vi "Teleop.vi"(10 "Match Info":T1={"Autonomous Elapsed Seconds"=0.0, "TeleOp Elapsed Seconds"=0.0, "Disabled Elapsed Seconds"=0.0, "Visited Autonomous"=FALSE, "Visited TeleOp"=FALSE, "Visited Disabled"=FALSE, "Autonomous Settings"={"Autonomous Style"=enum."Independent", "VI Refnum"=refnum}}, 11 "Call Context":T2) -> ()   [LabVIEW 2020]
doc: "This VI is called for each TeleOp packet received from the DS where the robot is not disabled. It is often used to read from the joysticks and update I/O or to update setpoints for timed control loops. It should complete and return within 20 milliseconds or it may miss DS packets."
uses:
  <vilib>/Rock Robotics/WPI/DriverStation/WPI_DriverStationDerivedRobotMode.ctl
  <vilib>/Rock Robotics/WPI/DriverStation/WPI_DriverStationMatch Info.ctl
  <vilib>/Rock Robotics/WPI/ThirdParty/Phoenix-LabVIEW/Motor Controller/Controls/CTRE_Phoenix_MotorControl_NeutralMode.ctl
  <vilib>/Rock Robotics/WPI/RobotDrive/WPI_RobotDriveDevRef.ctl
  <vilib>/Rock Robotics/WPI/MotorControl/WPI_MotorControlDeviceRef.ctl
  <vilib>/Rock Robotics/WPI/MotorControl/WPI_MotorControlType.ctl
  <vilib>/Rock Robotics/SystemInterfaces/DIO/FPGA_DIOPWMChannel.ctl
  <vilib>/Rock Robotics/WPI/PWM/WPI_PWMDeadband.ctl
  <vilib>/Rock Robotics/SystemInterfaces/DIO/FPGA_DIOChannel.ctl
  <vilib>/Rock Robotics/WPI/SafetyOutput/WPI_SafetyOutputConfigMenu.ctl
  <vilib>/Rock Robotics/WPI/Utilities/WPI_GetSetVariantRefNum.vi
  V1_nauru_2023_06_22/Global 1.vi
panel:
  out "FlagGarra":bool
  out "flagModoReto":bool
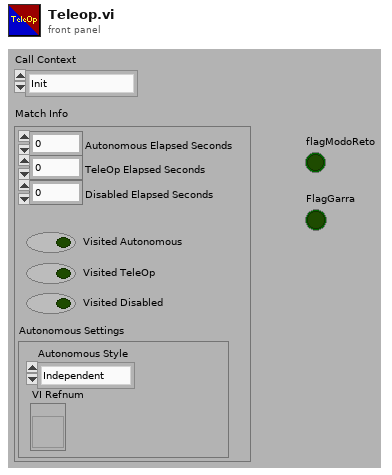
[diagram p1: front panel]
types:
  T1 = typedef "WPI_DriverStationMatch Info.ctl" = cluster{"Autonomous Elapsed Seconds":dbl, "TeleOp Elapsed Seconds":dbl, "Disabled Elapsed Seconds":dbl, "Visited Autonomous":bool, "Visited TeleOp":bool, "Visited Disabled":bool, "Autonomous Settings":cluster{"Autonomous Style":enum16{"Iterative", "Independent"}, "VI Refnum":refnum<vi>}}
  T2 = typedef "WPI_DriverStationDerivedRobotMode.ctl" = enum16{"Init", "Execute", "Stop"}
  T3 = typedef "WPI_SafetyOutputConfigMenu.ctl" = enum16{"Enable", "Disable"}
  T4 = typedef "WPI_RobotDriveDevRef.ctl" = cluster{"DevStatus":errorcluster, "Motors[]":T5[], "Square Inputs":bool, "Max Output":dbl}
  T5 = typedef "WPI_MotorControlDeviceRef.ctl" = cluster{"DeviceStatus":errorcluster, "Type":T6, "PWM":cluster{"PWM Channel":T7, "DeadBand":T8}, "CAN":cluster{"Device Number":u8, "SetOutput VI Ref":variant, "GetOutput VI Ref":variant, "Enable VI Ref":variant, "Disable VI Ref":variant, "Data":variant}, "Invert":bool, "DIO PWM":cluster{"PWM \"Enable\" Channel":T7, "DIOChannel":T9, "PWM Rate":dbl}}
  T6 = typedef "WPI_MotorControlType.ctl" = enum16{"PWM", "CAN", "DIO PWM"}
  T7 = typedef "FPGA_DIOPWMChannel.ctl" = enum8{"PWM 0", "PWM 1", "PWM 2", "PWM 3", "PWM 4", "PWM 5", "PWM 6", "PWM 7", "PWM 8", "PWM 9", "PWM MXP 0", "PWM MXP 1", "PWM MXP 2", "PWM MXP 3", "PWM MXP 4", "PWM MXP 5", "PWM MXP 6", "PWM MXP 7", "PWM MXP 8", "PWM MXP 9", "Invalid"}
  T8 = typedef "WPI_PWMDeadband.ctl" = cluster{"Name":string, "maxPositivePwm":i32, "minPositivePwm":i32, "centerPwm":i32, "maxNegativePwm":i32, "minNegativePwm":i32, "angularRange":u16}
  T9 = typedef "FPGA_DIOChannel.ctl" = enum8{"DIO 0", "DIO 1", "DIO 2", "DIO 3", "DIO 4", "DIO 5", "DIO 6", "DIO 7", "DIO 8", "DIO 9", "DIO MXP 0", "DIO MXP 1", "DIO MXP 2", "DIO MXP 3", "DIO MXP 4", "DIO MXP 5", "DIO MXP 6", "DIO MXP 7", "DIO MXP 8", "DIO MXP 9", "DIO MXP 10", "DIO MXP 11", "DIO MXP 12", "DIO MXP 13", "DIO MXP 14", "DIO MXP 15", "SPI Port CS1", "SPI Port CS2", "SPI Port CS3", "SPI Port MISO", "SPI Port MOSI", "Invalid"}
  T10 = typedef "CTRE_Phoenix_MotorControl_NeutralMode.ctl" = enum8{"EEPROMSetting", "Override to Coast", "Override to Brake"}
  T11 = typedef "WPI_JoystickDevRef.ctl" = cluster{"Device":T12}
  T12 = typedef "WPI_JoystickDeviceEnum.ctl" = enum16{"USB 0", "USB 1", "USB 2", "USB 3", "USB 4", "USB 5"}
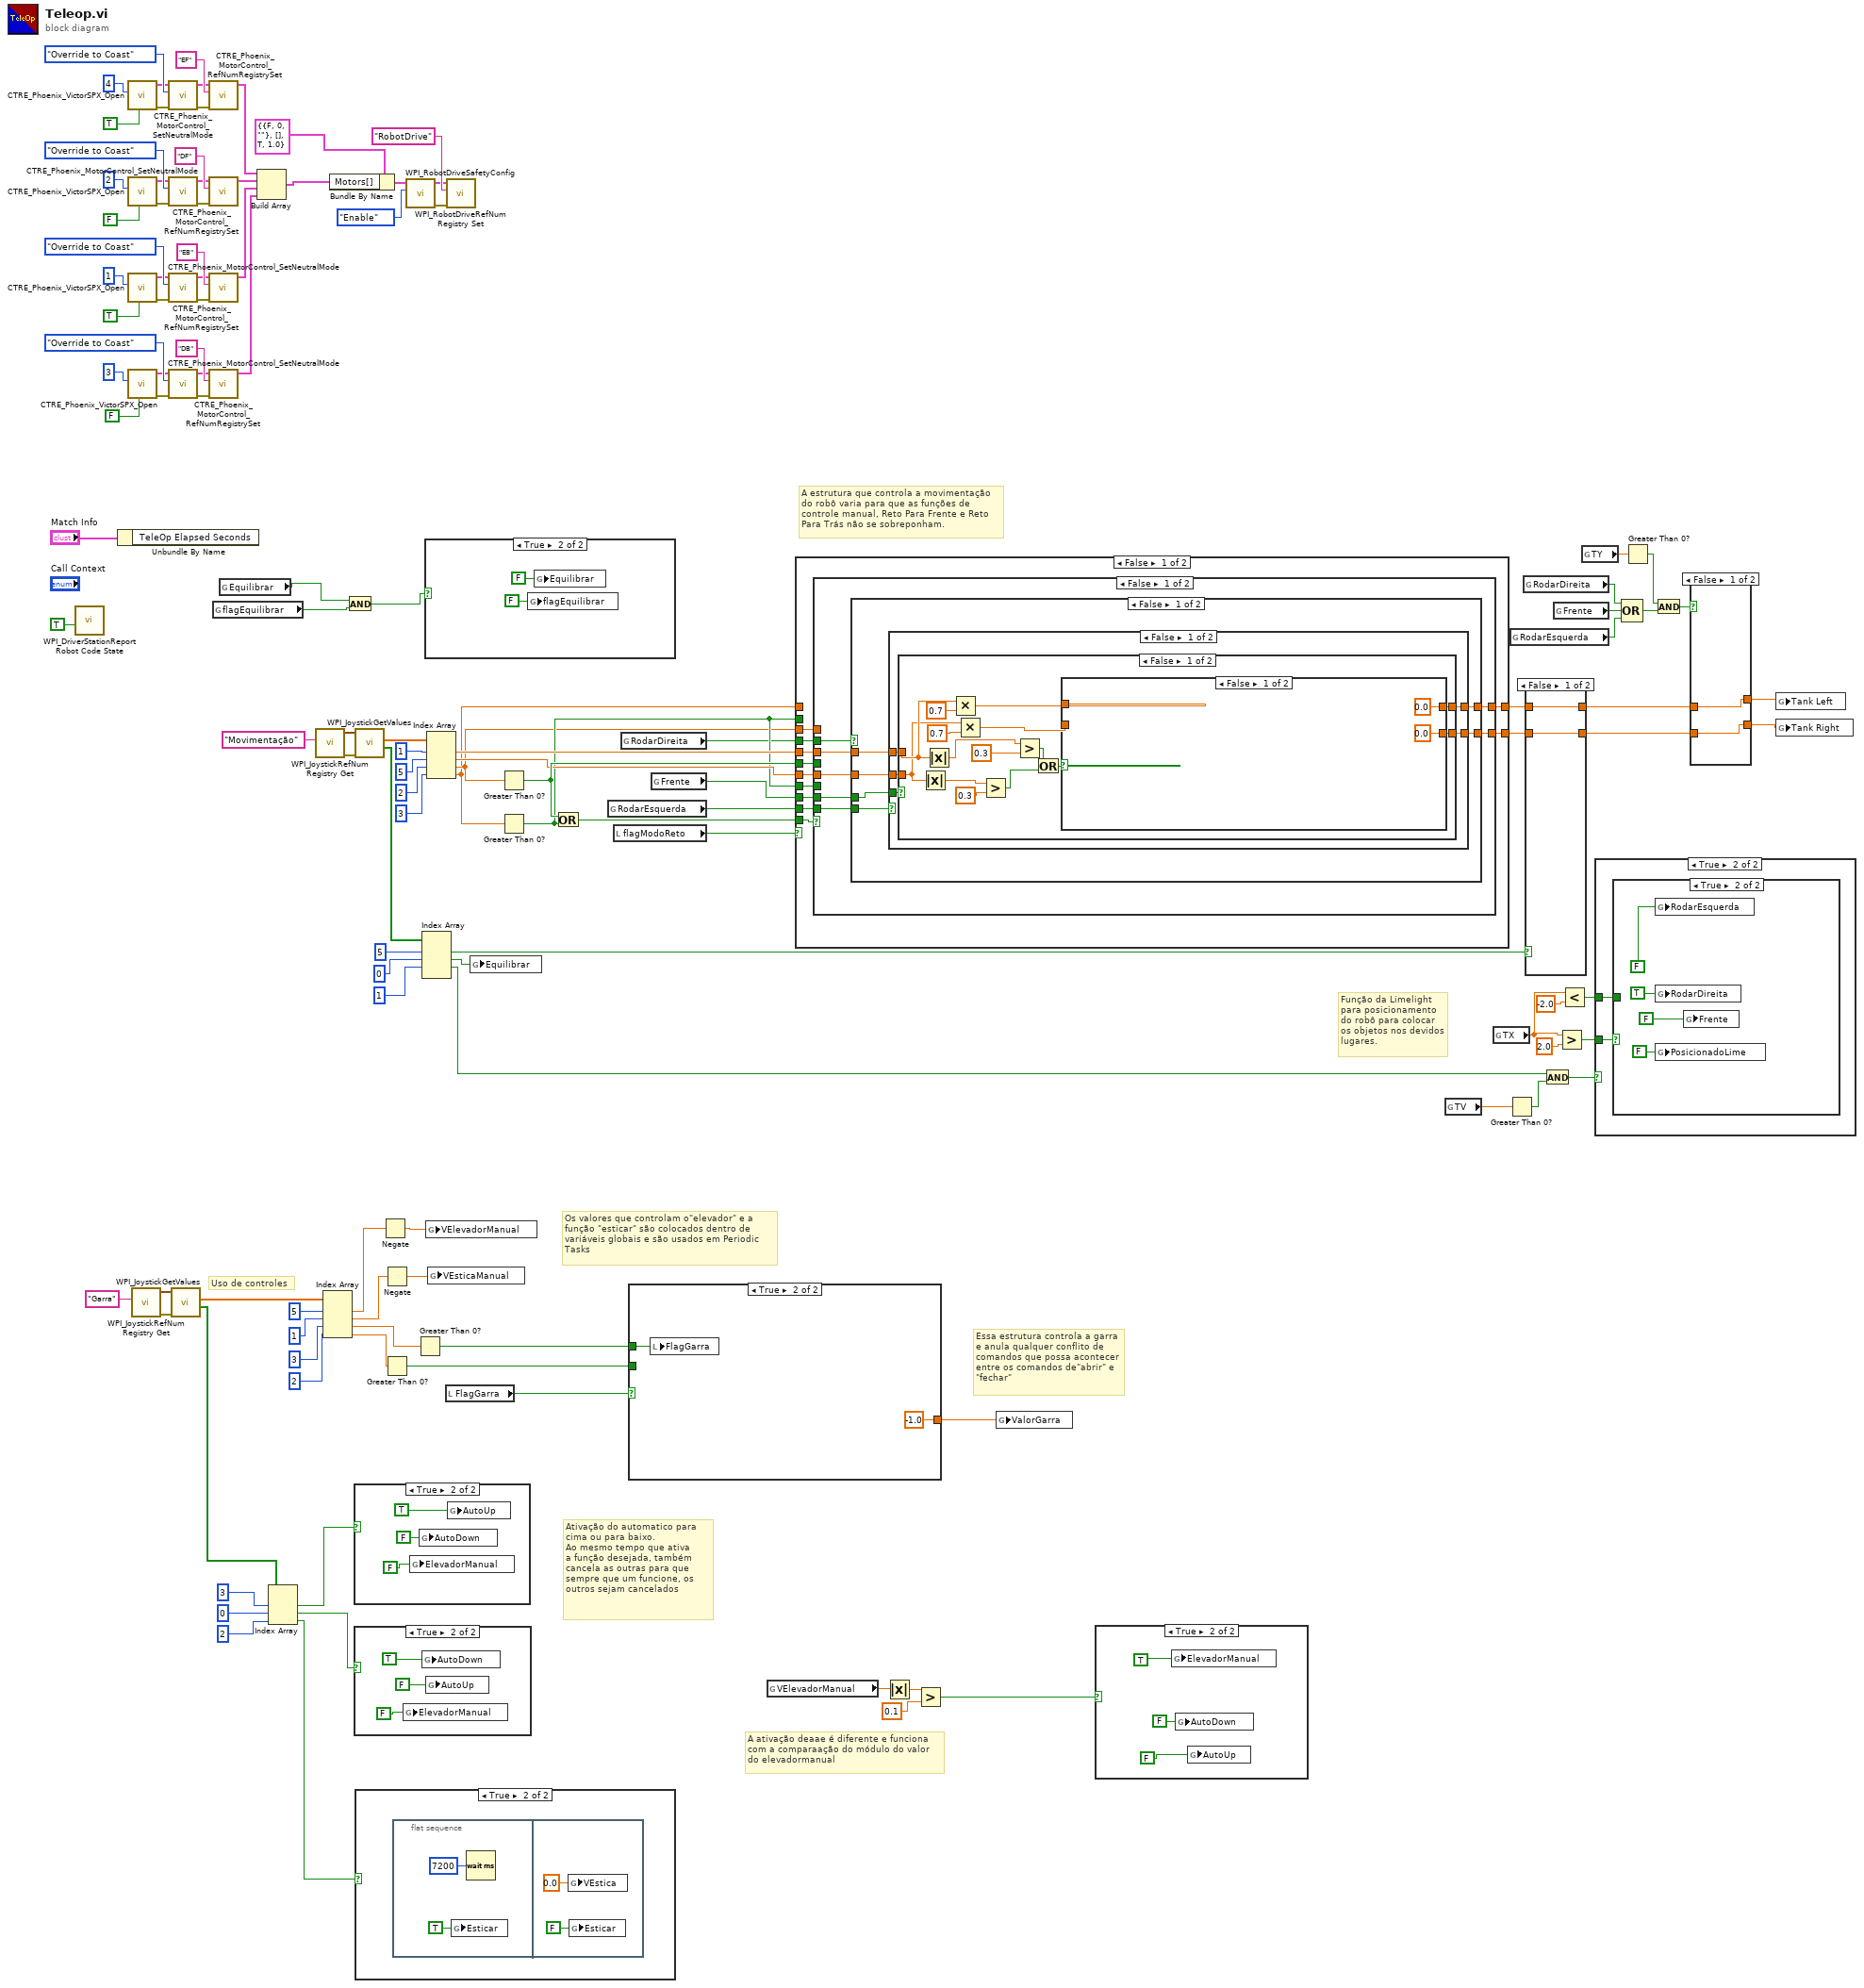
[diagram p0: block diagram]
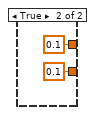
[diagram p4: hidden frame]
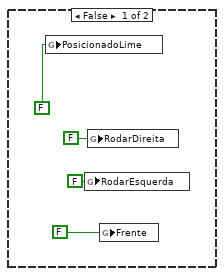
[diagram p5: hidden frame]
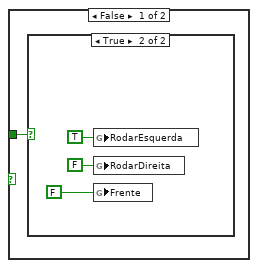
[diagram p6: hidden frame]
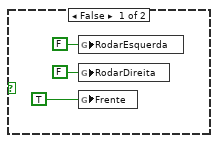
[diagram p7: hidden frame]
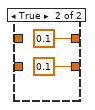
[diagram p8: hidden frame]
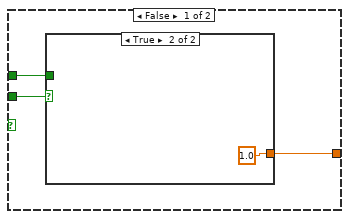
[diagram p12: hidden frame]
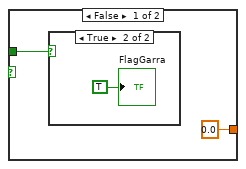
[diagram p13: hidden frame]
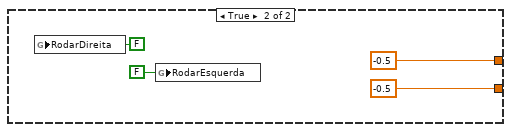
[diagram p16: hidden frame]
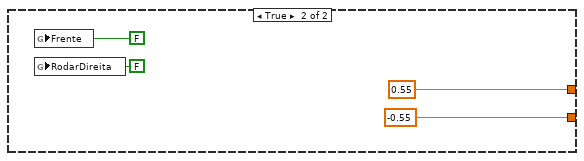
[diagram p17: hidden frame]
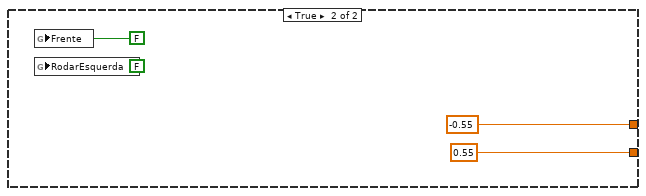
[diagram p18: hidden frame]
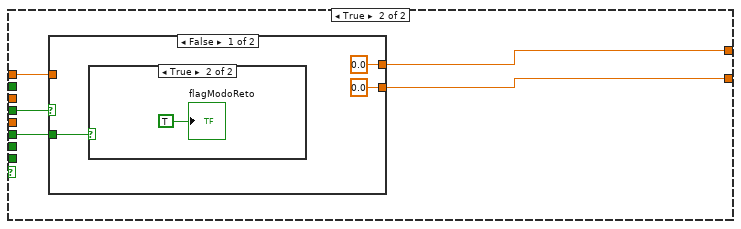
[diagram p19: hidden frame]
diagram:
  # "Função da Limelight para posicionamento do robô para colocar os objetos nos devidos lugares."
  # "Uso de controles"
  # "Essa estrutura controla a garra e anula qualquer conflito de comandos que possa acontecer entre os comandos de\"abrir\" e \"fechar\""
  # "Os valores que controlam o\"elevador\" e a função \"esticar\" são colocados dentro de variáveis globais e são usados em Periodic Tasks"
  # "A ativação deaae é diferente e funciona com a comparaação do módulo do valor do elevadormanual"
  # "A estrutura que controla a movimentação do robô varia para que as funções de controle manual, Reto Para Frente e Reto Para Trás não se sobreponham."
  # "Ativação do automatico para\ncima ou para baixo.\nAo mesmo tempo que ativa\na função desejada, também\ncancela as outras para que \nsempre que um funcione, os \noutros sejam cancelados"
  n1 = call <vilib>:"WPI_DriverStationReport Robot Code State.vi"("TeleOp"=TRUE ("Autonomous")) -> ()  [unwired: 10 in, 1 out]
  n2 = Unbundle By Name("Match Info") -> ()  [unwired: 1 out]
  n3 = call <vilib>:"CTRE_Phoenix_VictorSPX_Open.vi"("Invert"=TRUE, "Device Number"=u8 4) -> ("error out"=w8:errorcluster, "PhoenixMotorControlDevRef"=w9:T5)  [unwired: 8 in]
  n4 = call <vilib>:"CTRE_Phoenix_VictorSPX_Open.vi"("Invert"=FALSE, "Device Number"=u8 2) -> ("error out"=w16:errorcluster, "PhoenixMotorControlDevRef"=w17:T5)  [unwired: 8 in]
  n5 = call <vilib>:"CTRE_Phoenix_VictorSPX_Open.vi"("Invert"=TRUE, "Device Number"=u8 1) -> ("error out"=w24:errorcluster, "PhoenixMotorControlDevRef"=w25:T5)  [unwired: 8 in]
  n6 = call <vilib>:"CTRE_Phoenix_VictorSPX_Open.vi"("Invert"=FALSE, "Device Number"=u8 3) -> ("error out"=w32:errorcluster, "PhoenixMotorControlDevRef"=w33:T5)  [unwired: 8 in]
  n7 = call <vilib>:"WPI_JoystickRefNum Registry Get.vi"("refnum name"="Garra") -> ("error out"=w117:errorcluster, "JoystickDevRef"=w119:T11)  [unwired: 9 in]
  n8 = call <vilib>:"CTRE_Phoenix_MotorControl_SetNeutralMode.vi"("error in (no error)"=w8, "Motor Control Neutral Mode"=CTRE_Phoenix_MotorControl_NeutralMode."Override to Coast", "PhoenixMotorControlDevRef"=w9) -> ("error out"=w10:errorcluster, "PhoenixMotorControlDevRef"=w11:T5)  [unwired: 7 in]
  n9 = call <vilib>:"CTRE_Phoenix_MotorControl_SetNeutralMode.vi"("error in (no error)"=w16, "Motor Control Neutral Mode"=CTRE_Phoenix_MotorControl_NeutralMode."Override to Coast", "PhoenixMotorControlDevRef"=w17) -> ("error out"=w18:errorcluster, "PhoenixMotorControlDevRef"=w19:T5)  [unwired: 7 in]
  n10 = call <vilib>:"CTRE_Phoenix_MotorControl_SetNeutralMode.vi"("error in (no error)"=w24, "Motor Control Neutral Mode"=CTRE_Phoenix_MotorControl_NeutralMode."Override to Coast", "PhoenixMotorControlDevRef"=w25) -> ("error out"=w26:errorcluster, "PhoenixMotorControlDevRef"=w27:T5)  [unwired: 7 in]
  n11 = call <vilib>:"CTRE_Phoenix_MotorControl_SetNeutralMode.vi"("error in (no error)"=w32, "Motor Control Neutral Mode"=CTRE_Phoenix_MotorControl_NeutralMode."Override to Coast", "PhoenixMotorControlDevRef"=w33) -> ("error out"=w34:errorcluster, "PhoenixMotorControlDevRef"=w35:T5)  [unwired: 7 in]
  n12 = call <vilib>:"WPI_JoystickGetValues.vi"("error in (no error)"=w117, "JoystickDevRef"=w119) -> ("Buttons"=w122:bool[], "Axes"=w120:dbl[])  [unwired: 5 in, 3 out]
  n13 = call <vilib>:"CTRE_Phoenix_MotorControl_RefNumRegistrySet.vi"("error in (no error)"=w10, "refnum name"="EF", "PhoenixMotorControlDevRef"=w11) -> ("PhoenixMotorControlDevRef"=w40:T5)  [unwired: 7 in, 1 out]
  n14 = call <vilib>:"CTRE_Phoenix_MotorControl_RefNumRegistrySet.vi"("error in (no error)"=w18, "refnum name"="DF", "PhoenixMotorControlDevRef"=w19) -> ("PhoenixMotorControlDevRef"=w41:T5)  [unwired: 7 in, 1 out]
  n15 = call <vilib>:"CTRE_Phoenix_MotorControl_RefNumRegistrySet.vi"("error in (no error)"=w26, "refnum name"="EB", "PhoenixMotorControlDevRef"=w27) -> ("PhoenixMotorControlDevRef"=w42:T5)  [unwired: 7 in, 1 out]
  n16 = call <vilib>:"CTRE_Phoenix_MotorControl_RefNumRegistrySet.vi"("error in (no error)"=w34, "refnum name"="DB", "PhoenixMotorControlDevRef"=w35) -> ("PhoenixMotorControlDevRef"=w43:T5)  [unwired: 7 in, 1 out]
  n17 = global read "Global 1.vi" "flagEquilibrar"() -> (w54:bool)
  n18 = global read "Global 1.vi" "Equilibrar"() -> (w53:bool)
  n19 = Build Array(w40, w41, w42, w43) -> (w1:T5[])
  n20 = Index Array(array=w122, index #1=3 ("index"), index #2=0 ("index"), index #3=2 ("index")) -> (element #1=w95:bool, element #2=w94:bool, element #3=w44:bool)
  n21 = call <vilib>:"WPI_JoystickRefNum Registry Get.vi"("refnum name"="Movimentação") -> ("error out"=w114:errorcluster, "JoystickDevRef"=w115:T11)  [unwired: 9 in]
  n22 = Index Array(array=w120, index #1=5 ("index"), index #2=1 ("index"), index #3=3 ("index"), index #4=2 ("index")) -> (element #1=w87:dbl, element #2=w46:dbl, element #3=w47:dbl, element #4=w48:dbl)
  n23 = Bundle By Name(cluster=T4 {"DevStatus"={"status"=FALSE, "code"=0, "source"=""}, "Motors[]"=[], "Square Inputs"=TRUE, "Max Output"=1.0} ("RobotDriveDevRef"), "Motors[]"=w1) -> (w3:T4)
  n24 = And(x=w53, y=w54) -> (x .and. y?=w52:bool)
  n25 = case shown="True" w95 {
    frame False {
    }
    frame True {
      n26 = global write "Global 1.vi" "ElevadorManual"(FALSE ("ElevadorManual")) -> ()
      n27 = global write "Global 1.vi" "AutoDown"(FALSE ("AutoDown")) -> ()
      n28 = global write "Global 1.vi" "AutoUp"(TRUE ("AutoUp")) -> ()
    }
  }
  n29 = case shown="True" w94 {
    frame False {
    }
    frame True {
      n30 = global write "Global 1.vi" "ElevadorManual"(FALSE ("ElevadorManual")) -> ()
      n31 = global write "Global 1.vi" "AutoDown"(TRUE ("AutoDown")) -> ()
      n32 = global write "Global 1.vi" "AutoUp"(FALSE ("AutoDown")) -> ()
    }
  }
  n33 = call <vilib>:"WPI_JoystickGetValues.vi"("error in (no error)"=w114, "JoystickDevRef"=w115) -> ("Buttons"=w84:bool[], "Axes"=w113:dbl[])  [unwired: 5 in, 3 out]
  n34 = case shown="True" w44 {
    frame False {
    }
    frame True {
      n35 = flat-sequence {
        frame #0 {
          n36 = global write "Global 1.vi" "Esticar"(TRUE ("Retrair")) -> ()
          n37 = Wait (ms)(milliseconds to wait=u32 7200) -> ()  [unwired: 1 out]
        }
        frame #1 {
          n38 = global write "Global 1.vi" "VEstica"(0.0 ("VEstica")) -> ()
          n39 = global write "Global 1.vi" "Esticar"(FALSE ("Retrair")) -> ()
        }
      }
    }
  }
  n40 = Negate(x=w87) -> (-x=w88:dbl)
  n41 = Negate(x=w46) -> (-x=w45:dbl)
  n42 = Greater Than 0?(x=w48) -> (x > 0?=w100:bool)
  n43 = call <vilib>:"WPI_RobotDriveSafetyConfig.vi"("mode"=WPI_SafetyOutputConfigMenu."Enable", "RobotDriveDevRef"=w3) -> ("error out"=w5:errorcluster, "RobotDriveDevRef"=w6:T4)  [unwired: 2 in, 6 out]
  n44 = Greater Than 0?(x=w47) -> (x > 0?=w99:bool)
  n45 = Index Array(array=w84, index #1=5 ("index"), index #2=0 ("index"), index #3=1 ("index")) -> (element #1=w83:bool, element #2=w80:bool, element #3=w55:bool)  [unwired: 1 in, 1 out]
  n46 = case shown="True" w52 {
    frame False {
    }
    frame True {
      n47 = global write "Global 1.vi" "flagEquilibrar"(FALSE ("flagEquilibrar")) -> ()
      n48 = global write "Global 1.vi" "Equilibrar"(FALSE ("Equilibrar")) -> ()
    }
  }
  n49 = global write "Global 1.vi" "VElevadorManual"(w88) -> ()
  n50 = Index Array(array=w113, index #1=1 ("index"), index #2=5 ("index"), index #3=2 ("index"), index #4=3 ("index")) -> (element #1=w103:dbl, element #2=w102:dbl, element #3=w97:dbl, element #4=w96:dbl)
  n51 = global write "Global 1.vi" "VEsticaManual"(w45) -> ()
  n52 = local read "FlagGarra"() -> (w98:bool)
  n53 = call <vilib>:"WPI_RobotDriveRefNum Registry Set.vi"("error in (no error)"=w5, "refnum name"="RobotDrive", "RobotDriveDevRef"=w6) -> ()  [unwired: 7 in, 2 out]
  n54 = global write "Global 1.vi" "Equilibrar"(w80) -> ()
  n55 = Greater Than 0?(x=w97) -> (x > 0?=w105:bool)
  n56 = Greater Than 0?(x=w96) -> (x > 0?=w101:bool)
  n57 = Or(x=w105, y=w101) -> (x .or. y?=w106:bool)
  n58 = global read "Global 1.vi" "RodarEsquerda"() -> (w69:bool)
  n59 = local read "flagModoReto"() -> (w104:bool)
  n60 = global read "Global 1.vi" "RodarDireita"() -> (w70:bool)
  n61 = case shown="True" w98 {
    tunnel: w100 -> [w139 _]
    tunnel: w99 -> [w138 w144]
    tunnel: [w137 -1.0] -> w90
    frame False {
      n62 = case shown="True" w139 {
        tunnel: w138 -> [w141 _]
        tunnel: [0.0 1.0] -> w137
        frame False {
          n63 = case shown="True" w141 {
            frame False {
            }
            frame True {
              "FlagGarra" <- TRUE ("FlagGarra")
            }
          }
        }
        frame True {
        }
      }
    }
    frame True {
      n64 = local write "FlagGarra"(w144) -> ()
    }
  }
  n65 = global read "Global 1.vi" "Frente"() -> (w68:bool)
  n66 = global read "Global 1.vi" "VElevadorManual"() -> (w89:dbl)
  n67 = case shown="False" w104 {
    tunnel: w106 -> [w156 _]
    tunnel: w105 -> [w155 _]
    tunnel: w101 -> [w154 _]
    tunnel: w103 -> [w153 _]
    tunnel: w102 -> [w152 _]
    tunnel: [w151 w216] -> w86
    tunnel: [w150 w216] -> w85
    tunnel: w101 -> [_ w218]
    tunnel: w97 -> [w149 _]
    tunnel: w96 -> [_ w217]
    tunnel: w70 -> [w148 _]
    tunnel: w69 -> [w147 _]
    tunnel: w68 -> [w146 _]
    frame False {
      n68 = case shown="False" w156 {
        tunnel: w155 -> [_ w210]
        tunnel: w154 -> [_ w209]
        tunnel: w153 -> [w159 _]
        tunnel: w152 -> [w160 _]
        tunnel: [w157 w208] -> w151
        tunnel: [w158 w207] -> w150
        tunnel: w149 -> [_ w206]
        tunnel: w148 -> [w163 _]
        tunnel: w147 -> [w162 _]
        tunnel: w146 -> [w161 _]
        frame False {
          n69 = case shown="False" w163 {
            tunnel: w162 -> [w169 _]
            tunnel: w161 -> [w168 _]
            tunnel: w160 -> [w167 _]
            tunnel: w159 -> [w166 _]
            tunnel: [w165 -0.55] -> w157
            tunnel: [w164 0.55] -> w158
            frame False {
              n70 = case shown="False" w169 {
                tunnel: w168 -> [w174 _]
                tunnel: w167 -> [w173 _]
                tunnel: w166 -> [w172 _]
                tunnel: [w171 0.55] -> w165
                tunnel: [w170 -0.55] -> w164
                frame False {
                  n71 = case shown="False" w174 {
                    tunnel: w173 -> [w179 _]
                    tunnel: w172 -> [w180 _]
                    tunnel: [w182 -0.5] -> w171
                    tunnel: [w181 -0.5] -> w170
                    frame False {
                      n72 = Absolute Value(x=w179) -> (abs(x)=w189:dbl)
                      n73 = Absolute Value(x=w180) -> (abs(x)=w186:dbl)
                      n74 = Multiply(x=w180, y=0.7) -> (x*y=w176:dbl)
                      n75 = Multiply(x=w179, y=0.7) -> (x*y=w175:dbl)
                      n76 = Greater?(x=w189, y=0.3) -> (0:w184:bool)
                      n77 = Greater?(x=w186, y=0.3) -> (0:w185:bool)
                      n78 = Or(x=w185, y=w184) -> (x .or. y?=w183:bool)
                      n79 = case shown="False" w183 {
                        tunnel: w176 -> [_ w193]
                        tunnel: [0.0 w193] -> w182
                        tunnel: w175 -> [_ w192]
                        tunnel: [0.0 w192] -> w181
                        frame False {
                        }
                        frame True {
                        }
                      }
                    }
                    frame True {
                      n80 = global write "Global 1.vi" "RodarDireita"(FALSE ("RodarDireita")) -> ()
                      n81 = global write "Global 1.vi" "RodarEsquerda"(FALSE ("RodarDireita")) -> ()
                    }
                  }
                }
                frame True {
                  n82 = global write "Global 1.vi" "Frente"(FALSE ("RodarDireita")) -> ()
                  n83 = global write "Global 1.vi" "RodarDireita"(FALSE ("RodarDireita")) -> ()
                }
              }
            }
            frame True {
              n84 = global write "Global 1.vi" "Frente"(FALSE ("RodarDireita")) -> ()
              n85 = global write "Global 1.vi" "RodarEsquerda"(FALSE ("RodarDireita")) -> ()
            }
          }
        }
        frame True {
          n86 = case shown="False" w210 {
            tunnel: w209 -> [w213 _]
            tunnel: [0.0 w215] -> w208
            tunnel: [0.0 w215] -> w207
            tunnel: w206 -> [_ w215]
            frame False {
              n87 = case shown="True" w213 {
                frame False {
                }
                frame True {
                  "flagModoReto" <- TRUE ("flagModoReto")
                }
              }
            }
            frame True {
            }
          }
        }
      }
    }
    frame True {
      n88 = local write "flagModoReto"(w218) -> ()
      n89 = Negate(x=w217) -> (-x=w216:dbl)
    }
  }
  n90 = Absolute Value(x=w89) -> (abs(x)=w93:dbl)
  n91 = Greater?(x=w93, y=0.1) -> (0:w91:bool)
  n92 = global write "Global 1.vi" "ValorGarra"(w90) -> ()
  n93 = case shown="True" w91 {
    frame False {
    }
    frame True {
      n94 = global write "Global 1.vi" "ElevadorManual"(TRUE ("ElevadorManual")) -> ()
      n95 = global write "Global 1.vi" "AutoDown"(FALSE ("AutoDown")) -> ()
      n96 = global write "Global 1.vi" "AutoUp"(FALSE ("ElevadorManual")) -> ()
    }
  }
  n97 = global read "Global 1.vi" "TV"() -> (w71:dbl)
  n98 = global read "Global 1.vi" "TX"() -> (w76:dbl)
  n99 = Greater Than 0?(x=w71) -> (x > 0?=w73:bool)
  n100 = global read "Global 1.vi" "RodarEsquerda"() -> (w65:bool)
  n101 = global read "Global 1.vi" "RodarDireita"() -> (w67:bool)
  n102 = case shown="False" w83 {
    tunnel: [w222 0.1] -> w57
    tunnel: [w223 0.1] -> w58
    tunnel: w86 -> [w223 _]
    tunnel: w85 -> [w222 _]
    frame False {
    }
    frame True {
    }
  }
  n103 = And(x=w55, y=w73) -> (x .and. y?=w72:bool)
  n104 = global read "Global 1.vi" "Frente"() -> (w66:bool)
  n105 = Greater?(x=w76, y=2.0) -> (0:w75:bool)
  n106 = Less?(x=w76, y=-2.0) -> (x < y?=w78:bool)
  n107 = global read "Global 1.vi" "TY"() -> (w63:dbl)
  n108 = case shown="True" w72 {
    tunnel: w75 -> [_ w231]
    tunnel: w78 -> [_ w230]
    frame False {
      n109 = global write "Global 1.vi" "PosicionadoLime"(FALSE ("Posicionado")) -> ()
      n110 = global write "Global 1.vi" "RodarEsquerda"(FALSE ("RodarDireita")) -> ()
      n111 = global write "Global 1.vi" "RodarDireita"(FALSE ("RodarDireita")) -> ()
      n112 = global write "Global 1.vi" "Frente"(FALSE ("RodarEsquerda")) -> ()
    }
    frame True {
      n113 = case shown="True" w231 {
        tunnel: w230 -> [w232 _]
        frame False {
          n114 = case shown="True" w232 {
            frame False {
              n115 = global write "Global 1.vi" "RodarEsquerda"(FALSE ("RodarDireita")) -> ()
              n116 = global write "Global 1.vi" "RodarDireita"(FALSE ("RodarDireita")) -> ()
              n117 = global write "Global 1.vi" "Frente"(TRUE ("RodarEsquerda")) -> ()
            }
            frame True {
              n118 = global write "Global 1.vi" "RodarEsquerda"(TRUE ("RodarDireita")) -> ()
              n119 = global write "Global 1.vi" "RodarDireita"(FALSE ("RodarDireita")) -> ()
              n120 = global write "Global 1.vi" "Frente"(FALSE ("RodarEsquerda")) -> ()
            }
          }
        }
        frame True {
          n121 = global write "Global 1.vi" "RodarEsquerda"(FALSE ("RodarDireita")) -> ()
          n122 = global write "Global 1.vi" "RodarDireita"(TRUE ("RodarDireita")) -> ()
          n123 = global write "Global 1.vi" "PosicionadoLime"(FALSE ("Posicionado")) -> ()
          n124 = global write "Global 1.vi" "Frente"(FALSE ("RodarEsquerda")) -> ()
        }
      }
    }
  }
  n125 = Compound Arithmetic op=OR(w67, w66, w65) -> (w62:bool)
  n126 = Greater Than 0?(x=w63) -> (x > 0?=w64:bool)
  n127 = And(x=w64, y=w62) -> (x .and. y?=w61:bool)
  n128 = case shown="False" w61 {
    tunnel: [w244 0.1] -> w60
    tunnel: [w243 0.1] -> w59
    tunnel: w58 -> [w244 _]
    tunnel: w57 -> [w243 _]
    frame False {
    }
    frame True {
    }
  }
  n129 = global write "Global 1.vi" "Tank Left"(w60) -> ()
  n130 = global write "Global 1.vi" "Tank Right"(w59) -> ()
